vi "Operate.vi"(8 "Error In":errorcluster, 11 "Add In":refnum<class "Add.lvclass">) -> (0 "Error Out":errorcluster, 2 "C":dbl, 3 "Add Out":refnum<class "Add.lvclass">)   [LabVIEW 2021, in "Calculator.lvlib" / "Add.lvclass"]
doc: "This VI is an overriding method, which performs the addition operation."
uses:
  Add.lvclass
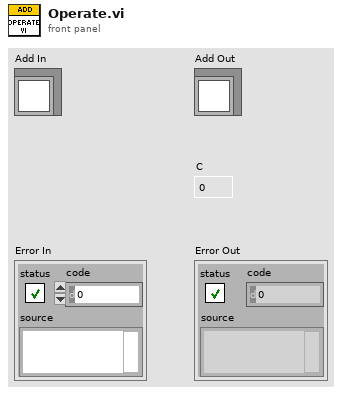
[diagram p1: front panel]
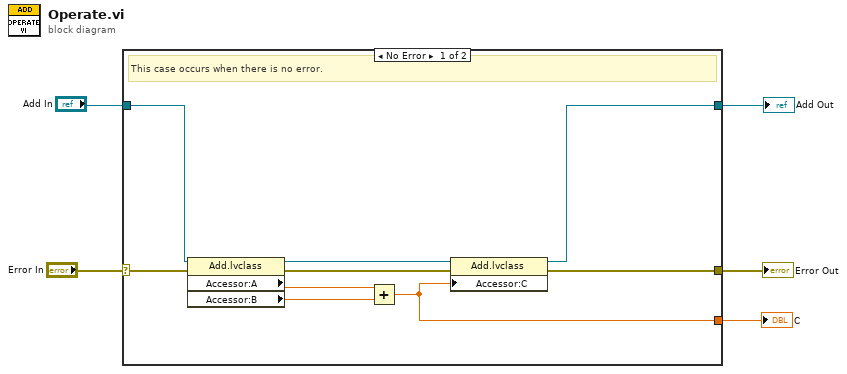
[diagram p0: block diagram]
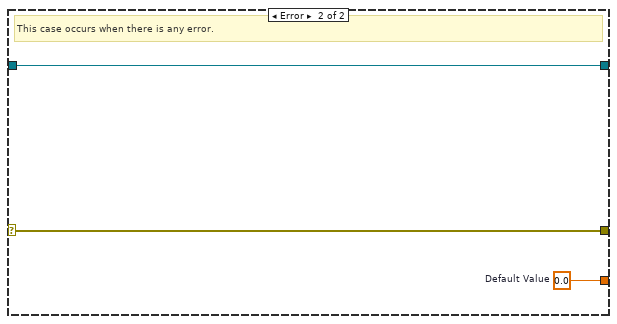
[diagram p2: hidden frame]
diagram:
  n1 = case shown="No Error" "Error In" {
    selector: "Error In" -> [w14 w17]
    tunnel: [w10 w17] -> w4
    tunnel: [w7 w16] -> w2
    tunnel: "Add In" -> [w6 w16]
    tunnel: [w8 w15] -> w1
    frame No Error {
      # "This case occurs when there is no error."
      n2 = property class="Add.lvclass"(reference=w6, error in=w14) -> (reference out=w9:refnum<class "Add.lvclass">, error out=w13:errorcluster, "Accessor:A"=w12:dbl, "Accessor:B"=w11:dbl)
      n3 = Add(x=w12, y=w11) -> (x+y=w8:dbl)
      n4 = property class="Add.lvclass"(reference=w9, error in=w13, "Accessor:C"=w8) -> (reference out=w7:refnum<class "Add.lvclass">, error out=w10:errorcluster)
    }
    frame Error {
      w15 = 0.0  # Default Value
      # "This case occurs when there is any error."
    }
  }
  "Error Out" <- w4
  "Add Out" <- w2
  "C" <- w1
